vi "Write OCP_Mode.vi"(8 "error in":errorcluster, 10 "OCP Mode":T1, 11 "89XX in":refnum<class "89XX.lvclass">) -> (0 "error out":errorcluster, 3 "89XX out":refnum<class "89XX.lvclass">)   [LabVIEW 2019, in "89XX.lvlib" / "89XX.lvclass"]
uses:
  Library/89XX.lvclass
  C:/Users/Public/Documents/Development/builds/Engine/Monitored Actor.lvlibp/Monitored Actor/Monitored Actor/Monitored Actor.lvclass
  builds/Instruments/PowerSupply.lvlibp/Custom Controls/OCP Mode.ctl
  builds/Engine/Monitored Actor.lvlibp/Monitored Actor/Monitored Actor/Read Actor Label.vi
  builds/Instruments/PowerSupply.lvlibp/Library/PowerSupply.lvclass
  <vilib>/ErrorRing/Error Ring.xnode
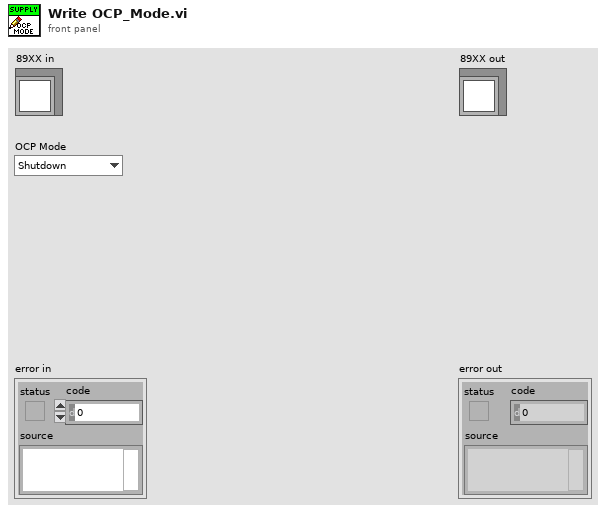
[diagram p1: front panel]
types:
  T1 = typedef "PowerSupply.lvlibp/PowerSupply.lvclass/OCP Mode.ctl" = enum16{"Shutdown", "Foldback"}
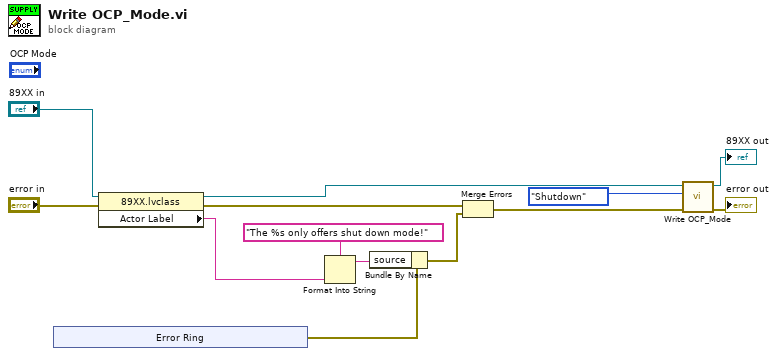
[diagram p0: block diagram]
diagram:
  n1 = xnode "Error Ring"() -> ("error out"=w10:errorcluster)
  n2 = property class="89XX.lvclass"(reference="89XX in", error in="error in") -> (reference out=w3:refnum<class "89XX.lvclass">, error out=w11:errorcluster, "Actor Label"=w7:string)
  n3 = Format Into String(format string="The %s only offers shut down mode!", w7) -> (resulting string=w9:string)  [unwired: 2 in, 1 out]
  n4 = Bundle By Name(cluster=w10, "source"=w9) -> (w8:errorcluster)
  n5 = Merge Errors(w11, w8) -> (w1:errorcluster)
  n6 = call-parent "Write OCP_Mode.vi"("error in"=w1, "OCP Mode"=OCP_Mode."Shutdown", "PowerSupply in"=w3) -> ("error out"=→"error out":errorcluster, "PowerSupply out"=→"89XX out":refnum<class "89XX.lvclass">)  [unwired: 7 in]
